vi "ConnectionString_AdminInfo(SubVI).vi"() -> (3 "ConnectionString":string)   [LabVIEW 2013]
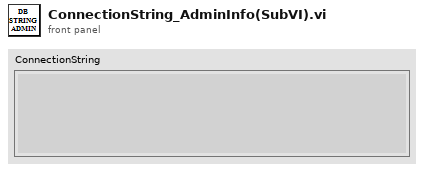
[diagram p1: front panel]
types:
  T1 = enum32{"invalid app kind", "Development System", "Run Time System", "Student Edition", "Embedded LabVIEW", "Evaluation", "Custom"}
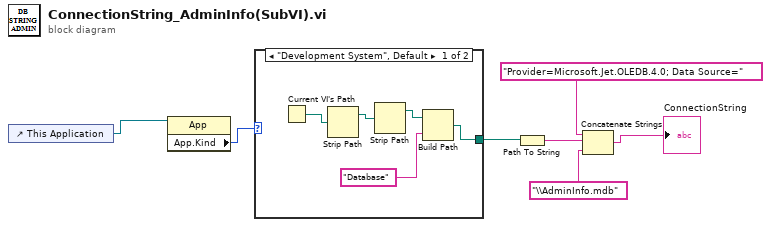
[diagram p0: block diagram]
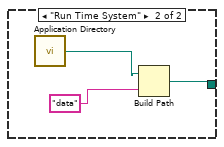
[diagram p2: hidden frame]
diagram:
  n1 = control-ref of="This Application"() -> (w7:refnum<vi>)
  n2 = property class="App"(reference=w7) -> ("App.Kind"=w6:T1)  [unwired: 1 in, 2 out]
  n3 = case shown="\"Development System\", Default" w6 {
    tunnel: [w11 w13] -> w2
    frame "Development System", Default {
      n4 = Current VI's Path() -> (path=w9:path)
      n5 = Strip Path(path=w9) -> (stripped path=w8:path)  [unwired: 1 out]
      n6 = Strip Path(path=w8) -> (stripped path=w12:path)  [unwired: 1 out]
      n7 = Build Path(base path=w12, name or relative path="Database") -> (appended path=w11:path)
    }
    frame "Run Time System" {
      n8 = call <vilib>:"Application Directory.vi"() -> ("Application Directory"=w15:path)
      n9 = Build Path(base path=w15, name or relative path="data") -> (appended path=w13:path)
    }
  }
  n10 = Path To String(path=w2) -> (string=w1:string)
  n11 = Concatenate Strings("Provider=Microsoft.Jet.OLEDB.4.0; Data Source=", w1, "\\AdminInfo.mdb") -> (→"ConnectionString":string)
